vi "Robot Main.vi"() -> ()   [LabVIEW 2017]
doc: "Robot Main serves as the primary scheduler for your command and control robotics program. It should not be necessary to modify this VI. Instead, you should add your code to the VIs called from Robot Main - Teleop, Autonomous, and SubSystems."
uses:
  <vilib>/Rock Robotics/WPI/Camera/WPI_CameraImageSize.ctl
  Support Code/Gyro/Gyro_TypeDef.ctl
  CtrlRefs/JoyStick2ALB.ctl
  CtrlRefs/JoyStick1ALB.ctl
  CtrlRefs/JoyStick2ALB(Analog).ctl
  CtrlRefs/JoyStick1ALV(Analog).ctl
  CtrlRefs/DioDisplayALB.ctl
  <vilib>/Rock Robotics/SystemInterfaces/NetworkCommunication/NetComm_UsageReport_ResourceType.ctl
  Framework/Robot Global Data.vi
  <vilib>/Rock Robotics/Network Tables/NT Write Number.vi
  Globals/Elapsed Time Global.vi
panel:
  in  "Tab Control":T1(tab)
  out "exeTime":u32(graph)
  out "CPU 0":dbl(graph)
  out "CPU 1":dbl(graph)
  out "Gyro_Data":T2
  out "J1 buttons":T3
  out "J2 buttons":T4
  out "Axes out 2":T5 {"Switch" format="%#_4g"; "Axis 2" format="%#_4g"; "Axis 1" format="%#_4g"; "Axis 0" format="%#_4g"}
  out "Axes out":T6 {"Slider" format="%#_4g"; "Axis 2" format="%#_4g"; "Axis 1" format="%#_4g"; "Axis 0" format="%#_4g"}
  out "DI out":T7
  in  "Image Size":T8=enum."320x240"
  in  "Enable Vision":bool
  in  "Finish":bool
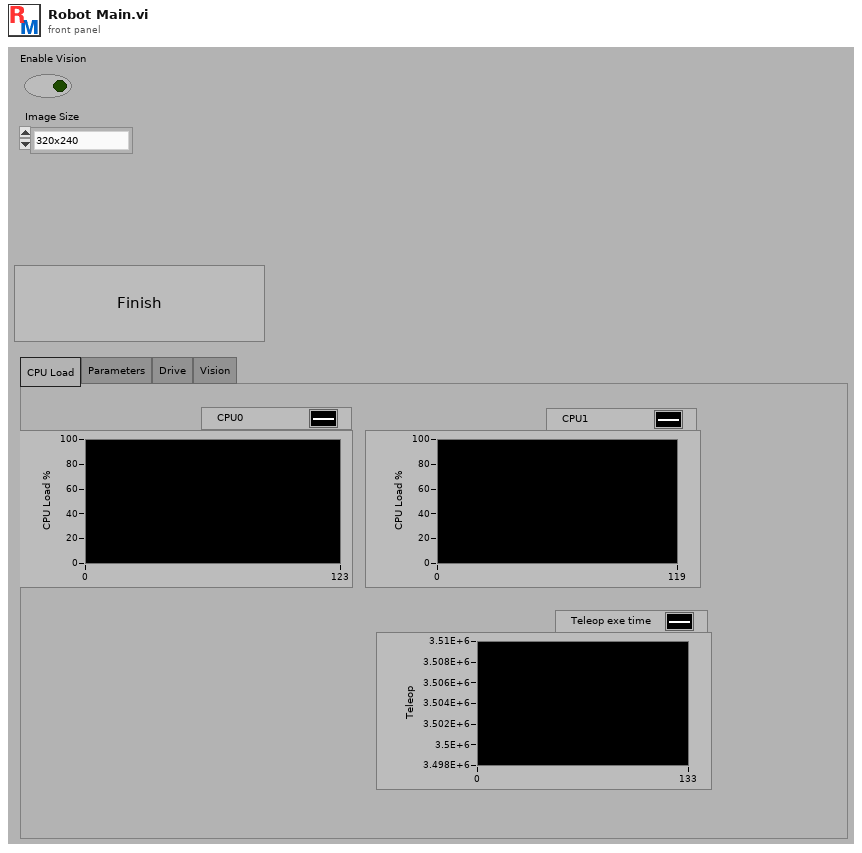
[diagram p1: front panel]
types:
  T1 = enum32{"CPU Load", "Parameters", "Drive", "Vision"}
  T2 = typedef "Gyro_TypeDef.ctl" = cluster{"Angle":dbl, "AngularRate":dbl, "Calibrated":bool}
  T3 = typedef "JoyStick1ALB.ctl" = cluster{"J1-B0":bool, "J1-B1":bool, "J1-B2":bool, "J1-B3":bool, "J1-B4":bool, "J1-B5":bool, "J1-B6":bool, "J1-B7":bool, "J1-B8-":bool, "J1-B9":bool, "J1-B10":bool, "J1-B11":bool}
  T4 = typedef "JoyStick2ALB.ctl" = cluster{"J2-B0":bool, "J2-B1":bool, "J2-B2":bool, "J2-B3":bool, "J2-B4":bool, "J2-B5":bool, "J2-B6":bool, "J2-B7":bool, "J2-B8":bool, "J2-B9":bool, "J2-B10":bool, "J2-B11":bool}
  T5 = typedef "JoyStick2ALB(Analog).ctl" = cluster{"Axis 0":dbl, "Axis 1":dbl, "Axis 2":dbl, "Switch":dbl}
  T6 = typedef "JoyStick1ALV(Analog).ctl" = cluster{"Axis 0":dbl, "Axis 1":dbl, "Axis 2":dbl, "Slider":dbl}
  T7 = typedef "DioDisplayALB.ctl" = cluster{"DIO 0-LiftMinLimitSwitch":bool, "DIO 1-LiftMaxLimitSwitch":bool, "DIO 2-LiftArmMinLimitSwitch":bool, "DIO 3-LiftArmMaxLimitSwitch":bool, "DIO 4-RightArmMaxLimitSwitch":bool, "DIO 5-RightArmMinLimitSwitch":bool, "DIO 6-LeftArmMaxLimitSwitch":bool, "DIO 7-LeftArmMinLimitSwitch":bool, "DIO 8":bool, "DIO 9":bool}
  T8 = typedef "WPI_CameraImageSize.ctl" = enum16{"640x480", "320x240", "160x120", "Custom"}
  T9 = typedef "NetComm_UsageReport_ResourceType.ctl" = enum8{"Controller", "Module", "Language", "CANPlugin", "Accelerometer", "ADXL345", "AnalogChannel", "AnalogTrigger", "AnalogTriggerOutput", "CANJaguar", "Compressor", "Counter", "Dashboard", "DigitalInput", "DigitalOutput", "DriverStationCIO", "DriverStationEIO", "DriverStationLCD", "Encoder", "GearTooth", "Gyro", "I2C", "Framework", "Jaguar", "Joystick", "Kinect", "KinectStick", "PIDController", "Preferences", "PWM", "Relay", "RobotDrive", "SerialPort", "Servo", "Solenoid", "SPI", "Task", "Ultrasonic", "Victor", "Button", "Command", "AxisCamera", "PCVideoServer", "SmartDashboard", "Talon", "HiTechnicColorSensor", "HiTechnicAccel", "HiTechnicCompass", "SRF08", "AnalogOutput", "Victor SP", "Talon SRX", "CAN Talon SRX", "ADXL362 Accel", "ADXRS450 Gyro", "Rev SPARK", "Mindsensors SD540", "Digital Filter", "ADIS16448", "PDP", "PCM", "PigeonIMU", "Nidec Brushless", "CTRE CANifier", "CTRE Future 0", "CTRE Future 1", "CTRE Future 2", "CTRE Future 3", "CTRE Future 4", "CTRE Future 5", "CTRE Future 6"}
  T10 = typedef "WPI_DriverStationMatch Info.ctl" = cluster{"Autonomous Elapsed Seconds":dbl, "TeleOp Elapsed Seconds":dbl, "Disabled Elapsed Seconds":dbl, "Visited Autonomous":bool, "Visited TeleOp":bool, "Visited Disabled":bool, "Autonomous Settings":cluster{"Autonomous Style":enum16{"Iterative", "Independent"}, "VI Refnum":refnum<vi>}}
  T11 = typedef "WPI_DriverStationDerivedRobotMode.ctl" = enum16{"Init", "Execute", "Stop"}
  T12 = typedef "WPI_DriverStationRobotMode2.ctl" = enum16{"Autonomous Disabled", "Autonomous Enabled", "Teleop Disabled", "Teleop Enabled", "Disconnected", "Finish", "Test Disabled", "Test Enabled", "Emergency Stopped"}
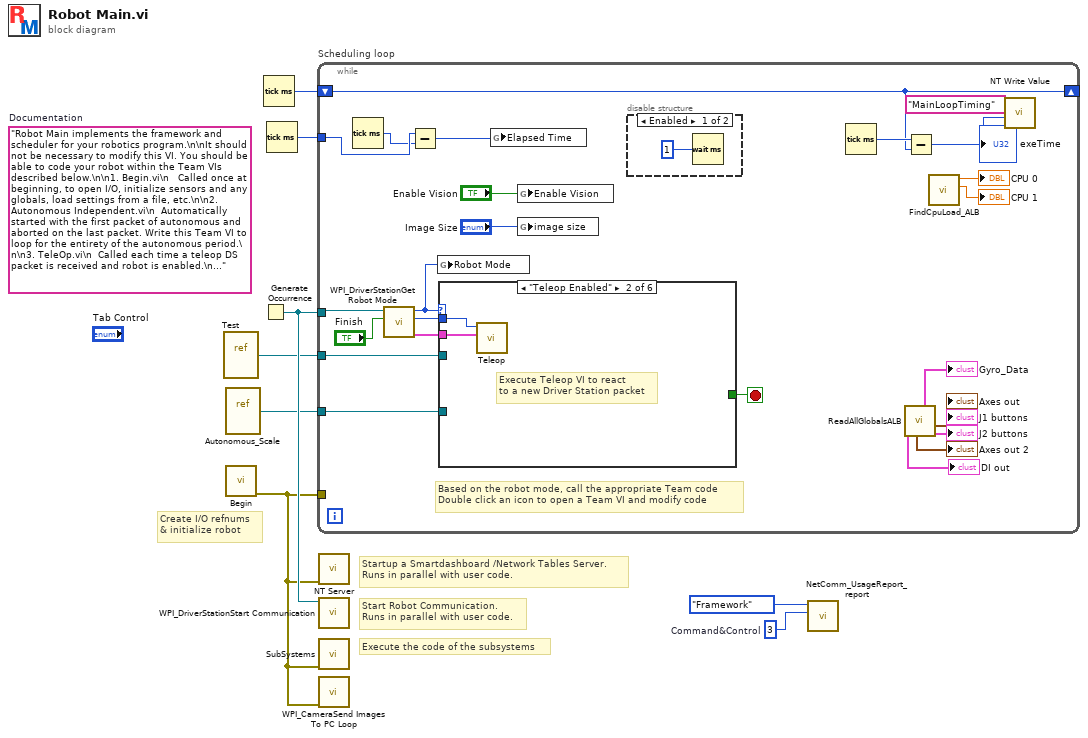
[diagram p0: block diagram]
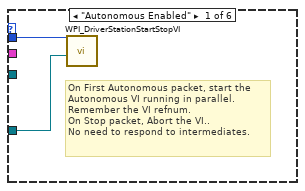
[diagram p3: hidden frame]
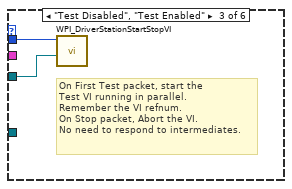
[diagram p4: hidden frame]
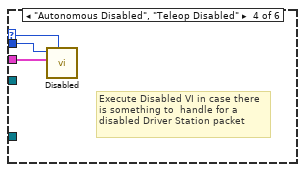
[diagram p5: hidden frame]
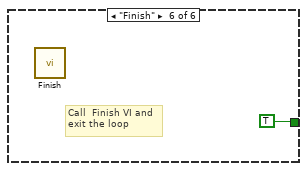
[diagram p7: hidden frame]
diagram:
  w4 = u8 3  # Command&Control
  (unwired) "Robot Main implements the framework and scheduler for your robotics program.\n\nIt should not be necessary to modify this VI. You should be able to code your robot within the Team VIs described below.\n\n1. Begin.vi\n   Called once at beginning, to open I/O, initialize sensors and any globals, load settings from a file, etc.\n\n2. Autonomous Independent.vi\n  Automatically started with the first packet of autonomous and aborted on the last packet. Write this Team VI to loop for the entirety of the autonomous period.\n\n3. TeleOp.vi\n  Called each time a teleop DS packet is received and robot is enabled.\n\n4. Disabled.vi\n  Called each time a packet is received and the robot is disabled.\n\n5. Test.vi\n  Called Automatically started with the first test packet and aborted on the last. Modify this VI to carry out robot and sensor validation tests.\n\n6. Vision.vi\n  A parallel loop that acquires and processes camera images.\n\n7. PeriodicTasks.vi\n  Parallel loops running at user-defined rates.\n\n8. Finish.vi\n  Called before exiting, so you can save data, clean up I/O, etc.\n"  # Documentation
  # "Startup a Smartdashboard /Network Tables Server.\nRuns in parallel with user code."
  # "Execute the code of the subsystems"
  # "Create I/O refnums\n& initialize robot"
  # "Start Robot Communication.\nRuns in parallel with user code."
  n1 = vi-ref "Test.vi"() -> (w6:refnum<vi>)
  n2 = vi-ref "Autonomous_Scale.vi"() -> (w7:refnum<vi>)
  n3 = call "Begin.vi"() -> ("error out"=w3:errorcluster)  [unwired: 2 in, 9 out]
  n4 = Generate Occurrence() -> (w8:refnum<k4>)
  n5 = Tick Count (ms)() -> (millisecond timer value=w2:u32)
  n6 = Tick Count (ms)() -> (millisecond timer value=w1:u32)
  n7 = while "Scheduling loop" {
    tunnel: w8 -> [w32]
    tunnel: w3 -> [_]
    tunnel: w7 -> [w27]
    tunnel: w6 -> [w25]
    shift-right: [w20] -> _
    shift-left: w2 -> [w20]
    tunnel: w1 -> [w11]
    stop <- w29 stop-if-true
    # "Based on the robot mode, call the appropriate Team code\nDouble click an icon to open a Team VI and modify code"
    n8 = Tick Count (ms)() -> (millisecond timer value=w10:u32)
    n9 = call <vilib>:"WPI_DriverStationGet Robot Mode.vi"("Finish"="Finish", "DS Occurrence"=w32) -> ("Match Info out"=w30:T10, "Call Context"=w33:T11, "Robot Mode"=w24:T12)  [unwired: 7 out]
    n10 = Subtract(x=w11, y=w10) -> (x-y=w9:u32)
    n11 = global write "Robot Global Data.vi" "Robot Mode"(w24) -> ()
    n12 = case shown="\"Teleop Enabled\"" w24 {
      selector: w24 -> [_ _ _ w41 _ _]
      tunnel: w33 -> [w36 w38 w40 w43 _ _]
      tunnel: w30 -> [_ w37 _ w42 _ _]
      tunnel: [_ _ _ _ _ TRUE] -> w29
      tunnel: w27 -> [w35 _ _ _ _ _]
      tunnel: w25 -> [_ _ w39 _ _ _]
      frame "Autonomous Enabled" {
        # "On First Autonomous packet, start the\nAutonomous VI running in parallel.\nRemember the VI refnum.\nOn Stop packet, Abort the VI..\nNo need to respond to intermediates."
        n13 = call <vilib>:"WPI_DriverStationStartStopVI.vi"("VI in"=w35, "Call Context"=w36) -> ()  [unwired: 10 in]
      }
      frame "Teleop Enabled" {
        # "Execute Teleop VI to react\nto a new Driver Station packet"
        n14 = call "Teleop.vi"("Match Info"=w37, "Call Context"=w38) -> ()  [unwired: 1 in, 9 out]
      }
      frame "Test Disabled", "Test Enabled" {
        # "On First Test packet, start the\nTest VI running in parallel.\nRemember the VI refnum.\nOn Stop packet, Abort the VI.\nNo need to respond to intermediates."
        n15 = call <vilib>:"WPI_DriverStationStartStopVI.vi"("VI in"=w39, "Call Context"=w40) -> ()  [unwired: 10 in]
      }
      frame "Autonomous Disabled", "Teleop Disabled" {
        # "Execute Disabled VI in case there\nis something to  handle for a\ndisabled Driver Station packet"
        n16 = call "Disabled.vi"("Robot Mode"=w41, "Match Info"=w42, "Call Context"=w43) -> ()  [unwired: 1 in, 8 out]
      }
      frame "Disconnected", Default {
        # "Driver Station packet didn't arrive.\nPossibly useful for diagnostics"
      }
      frame "Finish" {
        # "Call  Finish VI and\nexit the loop"
        n17 = call "Finish.vi"() -> ()  [unwired: 1 in, 7 out]
      }
    }
    n18 = global write "Elapsed Time Global.vi" "Elapsed Time"(w9) -> ()
    n19 = global write "Robot Global Data.vi" "Enable Vision"("Enable Vision") -> ()
    n20 = global write "Robot Global Data.vi" "image size"("Image Size") -> ()
    n21 = disable-structure shown="Enabled" {
      frame Enabled {
        n22 = Wait (ms)(milliseconds to wait=u32 1) -> ()  [unwired: 1 out]
      }
      frame Disabled {
      }
    }
    n23 = Tick Count (ms)() -> (millisecond timer value=w23:u32)
    n24 = call "ReadAllGlobalsALB.vi"() -> ("J1 buttons"=→"J1 buttons":T3, "Axes out"=→"Axes out":T6, "J2 buttons"=→"J2 buttons":T4, "Gyro_Data"=→"Gyro_Data":T2, "Axes out 2"=→"Axes out 2":T5, "DI out"=→"DI out":T7)  [unwired: 4 in, 2 out]
    n25 = Subtract(x=w23, y=w20) -> (x-y=w18:u32)
    "exeTime" <- w18
    n26 = call "FindCpuLoad_ALB.vi"() -> ("CPU2 out"=→"CPU 1":dbl, "CPU1 out"=→"CPU 0":dbl)  [unwired: 10 in]
    n27 = call-poly <vilib>:"NT Write Value.vi"("Numeric"=w18, "Name"="MainLoopTiming") -> ()  [unwired: 9 in, 1 out]
  }
  n28 = call <vilib>:"NT Server.vi"("error in (no error)"=w3) -> ()  [unwired: 11 in]
  n29 = call <vilib>:"WPI_DriverStationStart Communication.vi"("occurrence"=w8) -> ()  [unwired: 1 in, 10 out]
  n30 = call "SubSystems.vi"("error in"=w3) -> ()  [unwired: 11 in]
  n31 = call <vilib>:"WPI_CameraSend Images To PC Loop.vi"("error in (no error)"=w3) -> ()  [unwired: 11 in]
  n32 = call <vilib>:"NetComm_UsageReport_report.vi"("Instance Number"=w4, "Resource Type"=NetComm_UsageReport_ResourceType."Framework") -> ()  [unwired: 10 in]
